vi "Find Best Trending Stock.vi"(11 "Maximum Price":string) -> (3 "resulting prompt":string)   [LabVIEW 2020, in "Full Featured MCP Server.lvlib"]
doc: "Investigates current and past prices to detect best trending stocks. Ignores stocks above maximum price."
uses:
  Full Featured MCP Server.lvlib
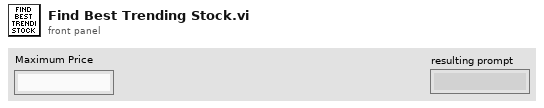
[diagram p1: front panel]
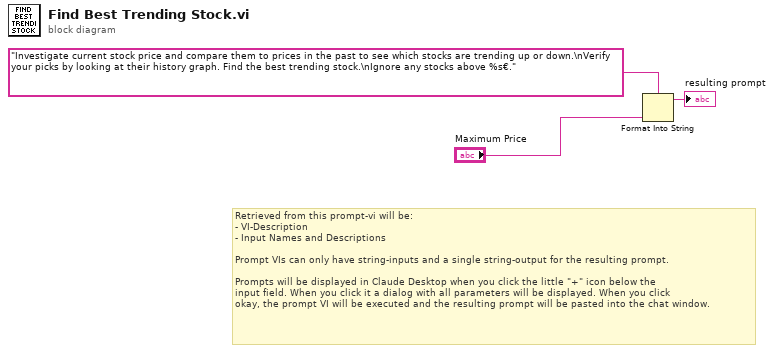
[diagram p0: block diagram]
diagram:
  # "Retrieved from this prompt-vi will be:\n- VI-Description\n- Input Names and Descriptions\n\nPrompt VIs can only have string-inputs and a single string-output for the resulting prompt.\n\nPrompts will be displayed in Claude Desktop when you click the little \"+\" icon below the \ninput field. When you click it a dialog with all parameters will be displayed. When you click\nokay, the prompt VI will be executed and the resulting prompt will be pasted into the chat window."
  n1 = Format Into String(format string="Investigate current stock price and compare them to prices in the past to see which stocks are trending up or down.\nVerify your picks by looking at their history graph. Find the best trending stock.\nIgnore any stocks above %s€.", "Maximum Price") -> (resulting string=→"resulting prompt":string)  [unwired: 2 in, 1 out]
